vi "__JSONtext__Variant to Flattened String (special).vi"(11 "Variant":variant) -> (1 "data":string, 2 "type":i16[](array[numeric]))   [LabVIEW 2017]
doc: "This VI was copied from JSONtext.\n\n---\n\nJSONtext\n\nCopyright 2017-21, JDP Science Limited\nAll rights reserved.\n\nRedistribution and use in source and binary forms, with or without\nmodification, are permitted provided that the following conditions are met: \n\n1. Redistributions of source code must retain the above copyright notice, this\n list of conditions and the following disclaimer. \n2. Redistributions in binary form must reproduce the following disclaimer in the\n documentation and/or other materials provided with the distribution. \n\nTHIS SOFTWARE IS PROVIDED BY THE COPYRIGHT HOLDERS AND CONTRIBUTORS \"AS IS\" AND\nANY EXPRESS OR IMPLIED WARRANTIES, INCLUDING, BUT NOT LIMITED TO, THE IMPLIED\nWARRANTIES OF MERCHANTABILITY AND FITNESS FOR A PARTICULAR PURPOSE ARE\nDISCLAIMED. IN NO EVENT SHALL THE COPYRIGHT OWNER OR CONTRIBUTORS BE LIABLE FOR\nANY DIRECT, INDIRECT, INCIDENTAL, SPECIAL, EXEMPLARY, OR CONSEQUENTIAL DAMAGES\n(INCLUDING, BUT NOT LIMITED TO, PROCUREMENT OF SUBSTITUTE GOODS OR SERVICES;\nLOSS OF USE, DATA, OR PROFITS; OR BUSINESS INTERRUPTION) HOWEVER CAUSED AND\nON ANY THEORY OF LIABILITY, WHETHER IN CONTRACT, STRICT LIABILITY, OR TORT\n(INCLUDING NEGLIGENCE OR OTHERWISE) ARISING IN ANY WAY OUT OF THE USE OF THIS\nSOFTWARE, EVEN IF ADVISED OF THE POSSIBILITY OF SUCH DAMAGE."
uses:
  <vilib>/Utility/Data Type/NI_Data Type.lvlib
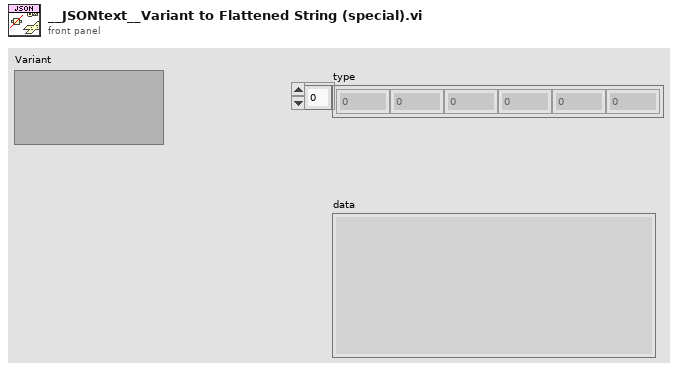
[diagram p1: front panel]
types:
  T1 = typedef "NI_Data Type.lvlib/Data Type.ctl" = enum8{"Invalid Type", "Void", "I8", "I16", "I32", "I64", "U8", "U16", "U32", "U64", "Single Float", "Double Float", "Extended Float", "Single Complex", "Double Complex", "Extended Complex", "Enum U8", "Enum U16", "Enum U32", "Enum U64", "Single Float With Unit", "Double Float With Unit", "Extended Float With Unit", "Single Complex with Unit", "Double Complex with Unit", "Extended Complex with Unit", "Boolean", "String", "Path", "Picture", "Tag", "Array", "Cluster", "Variant", "LV Variant", "Waveform", "Timestamp", "Digital Waveform", "Digital Data", "ExpressData", "Refnum", "External Data", "VI", "Poly VI", "LabVIEW Class Instance", "Fixed Point"}
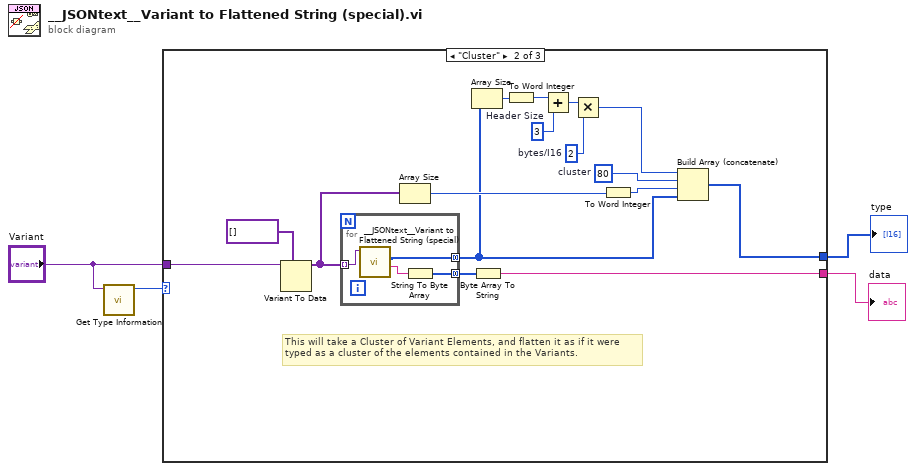
[diagram p0: block diagram]
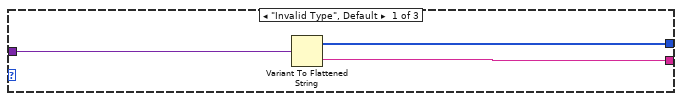
[diagram p2: hidden frame]
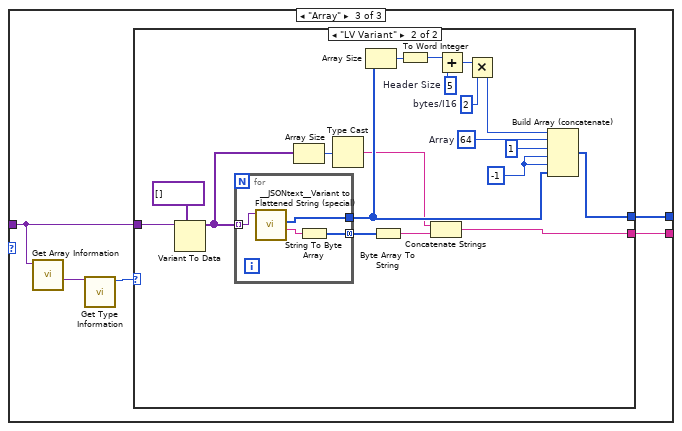
[diagram p3: hidden frame]
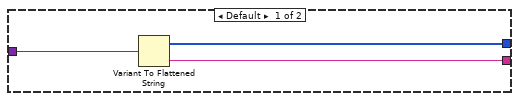
[diagram p4: hidden frame]
diagram:
  n1 = call <vilib>:"Get Type Information.vi"("Variant"="Variant") -> ("Type"=w4:T1)  [unwired: 6 in, 4 out]
  n2 = case shown="\"Cluster\"" w4 {
    tunnel: "Variant" -> [w7 w23 w30]
    tunnel: [w5 w9 w32] -> w1
    tunnel: [w6 w8 w31] -> w2
    frame "Invalid Type", Default {
      n3 = Variant To Flattened String(Variant=w7) -> (data string=w5:string, 1:w6:i16[])
    }
    frame "Cluster" {
      w12 = i16 80  # cluster
      w15 = i16 2  # bytes/I16
      w17 = i16 3  # Header Size
      # "This will take a Cluster of Variant Elements, and flatten it as if it were\ntyped as a cluster of the elements contained in the Variants."
      n4 = Variant To Data(type=variant[] [], Variant=w23) -> (data=w21:variant[])  [unwired: 1 in, 1 out]
      n5 = for {
        tunnel: w21 -> [w26] mode=indexing
        tunnel: [w27] -> w10 mode=concatenating
        tunnel: [w25] -> w11 mode=concatenating
        n6 = call "__JSONtext__Variant to Flattened String (special).vi"("Variant"=w26) -> ("data"=w24:string, "type"=w25:i16[])  [unwired: 9 in]
        n7 = String To Byte Array(string=w24) -> (unsigned byte array=w27:u8[])
      }
      n8 = Array Size(array=w21) -> (size(s)=w13:i32)
      n9 = Array Size(array=w11) -> (size(s)=w20:i32)
      n10 = Byte Array To String(unsigned byte array=w10) -> (string=w9:string)
      n11 = To Word Integer(number=w20) -> (16bit integer=w14:i16)
      n12 = Add(x=w14, y=w17) -> (x+y=w16:i16)
      n13 = Multiply(x=w16, y=w15) -> (x*y=w19:i16)
      n14 = To Word Integer(number=w13) -> (16bit integer=w18:i16)
      n15 = Build Array (concatenate)(w19, w12, w18, w11) -> (w8:i16[])
    }
    frame "Array" {
      n16 = call <vilib>:"Get Array Information.vi"("Variant"=w30) -> ("Array Element Data Type"=w29:variant)  [unwired: 7 in, 3 out]
      n17 = call <vilib>:"Get Type Information.vi"("Variant"=w29) -> ("Type"=w28:T1)  [unwired: 6 in, 4 out]
      n18 = case shown="\"LV Variant\"" w28 {
        tunnel: [w33 w38] -> w32
        tunnel: [w34 w42] -> w31
        tunnel: w30 -> [w35 w41]
        frame Default {
          n19 = Variant To Flattened String(Variant=w35) -> (data string=w33:string, 1:w34:i16[])
        }
        frame "LV Variant" {
          w36 = i16 -1 ("element")
          w46 = i16 64  # Array
          w48 = i16 2  # bytes/I16
          w50 = i16 5  # Header Size
          n20 = Variant To Data(type=variant[] [], Variant=w41) -> (data=w53:variant[])  [unwired: 1 in, 1 out]
          n21 = for {
            tunnel: w53 -> [w57] mode=indexing
            tunnel: [w58] -> w44 mode=concatenating
            tunnel: [w56] -> w45
            n22 = call "__JSONtext__Variant to Flattened String (special).vi"("Variant"=w57) -> ("data"=w55:string, "type"=w56:i16[])  [unwired: 9 in]
            n23 = String To Byte Array(string=w55) -> (unsigned byte array=w58:u8[])
          }
          n24 = Array Size(array=w53) -> (size(s)=w39:i32)
          n25 = Type Cast(x=w39) -> (*(type *) &x=w37:string)  [unwired: 1 in]
          n26 = Array Size(array=w45) -> (size(s)=w52:i32)
          n27 = Byte Array To String(unsigned byte array=w44) -> (string=w43:string)
          n28 = To Word Integer(number=w52) -> (16bit integer=w47:i16)
          n29 = Concatenate Strings(w37, w43) -> (w38:string)
          n30 = Add(x=w47, y=w50) -> (x+y=w49:i16)
          n31 = Multiply(x=w49, y=w48) -> (x*y=w51:i16)
          n32 = Build Array (concatenate)(w51, w46, i16 1 ("element"), w36, w36, w45) -> (w42:i16[])
        }
      }
    }
  }
  "type" <- w2
  "data" <- w1
